vi "Buffered Log String Indicator Example.vi"() -> ()   [LabVIEW 2019, in "Logger Examples.lvlib"]
uses:
  Logger Examples.lvlib
  Source/Composed Log/Types/Log Level.ctl
  Source/String Formats/String Expression Format/String Expression Format.lvclass/String Expression Format.ctl
  Source/Composed Log/LoggerReference/LoggerReference.lvclass/LoggerReference.ctl
  601d143e-8928-4a3b-9174-3083e729aaa9.vi
  Source/String Formats/String Expression Format/Run Formatter.vi
  Source/Composed Log/LoggerReference/Return Aggregate Queues.vi
  Source/Composed Log/LoggerReference/Add Aggregate Log.vi
  601d143e-8928-4a3b-9174-3083e729aaa9.vi/16370e4d-f3cd-41c1-a9a1-4fb3403731d5.vi
  Source/Composed Log/LoggerReference/Log.vi
  Source/Composed Log/LoggerReference/Get Valid Event Time.vi
  <vilib>/dlg_ctls.llb/Space Constant.vi
  Source/Composed Log/LoggerReference/Send Add Sink.vi
  Source/Composed Log/LoggerReference/Remove Stale Logs.vi
  Source/String Formats/String Expression Format/String Expression Format.lvclass
  C:/CS/Log/Source/IStringFormat/IStringFormat.lvclass
  Source/String Control Sink/String Control Sink.lvclass
  C:/CS/Log/Source/String Log Sink/String Log Sink.lvclass
  C:/CS/Log/Source/Composed Log/Log Sink/Log Sink.lvclass
  Source/Buffered String Log Sink/Buffered String Log Sink.lvclass
  Source/Composed Log/Application Logger/Launch Worker Loop.vi
  Source/Composed Log/LoggerReference/Initialize Logger Instance.vi
  Source/Composed Log/LoggerReference/LoggerReference.lvclass
  Source/Composed Log/IErrorFormat/IErrorFormat.lvclass
  Source/Composed Log/Log Sink/Log Sink.lvclass
  Source/Composed Log/Composed Log.lvlib
panel:
  in  "Log Error":bool
  in  "Error Information":string
  in  "Error Code":i32
  in  "Event Level":T1(ring)
  out "250ms Timeout, 128 Element Buffer":string
  out "No Timeout - 50 Element Buffer":string
  out "No Timeout, Unlimited Buffer":string
  in  "Data To Log":string
  in  "Source":string="User"
  in  "Log":bool
  # "This Sink will log events as they arrive, up until the buffer is full. After that, each new event will push out the oldest."
  # "This Sink will log every event as it arrives, and grow endlessly as the application is run."
  # "This Sink will only log events on a 250ms interval. Every 250ms, if new events are available, they will be pushed to the string. A fixed length buffer is also used - only the latest 128 events will be shown."
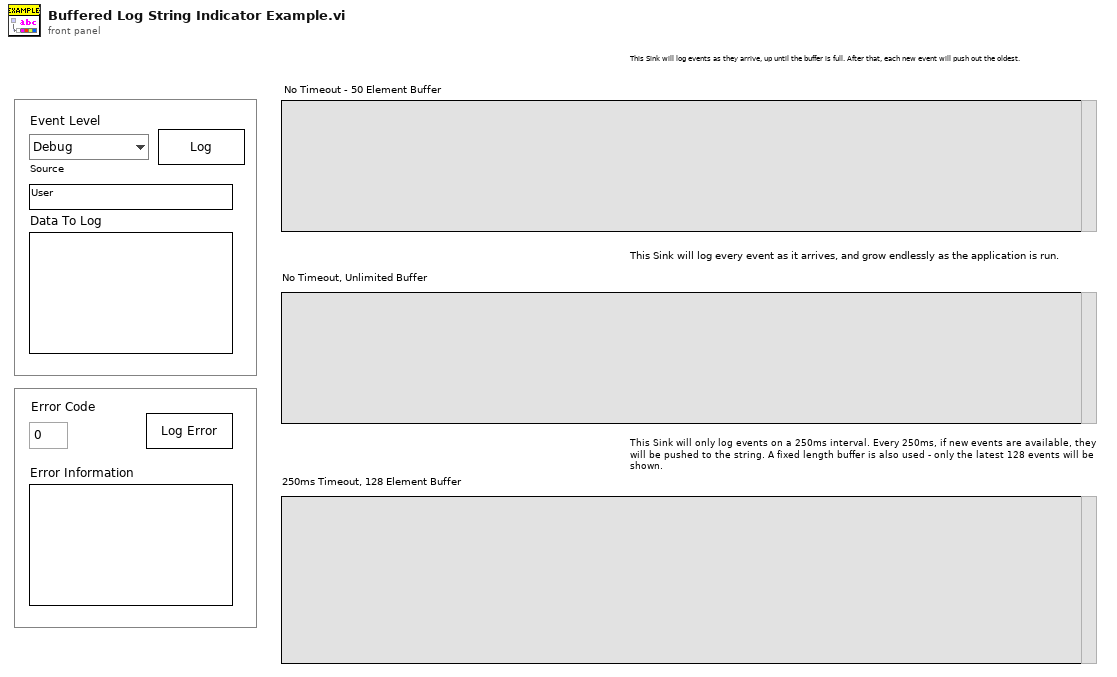
[diagram p1: front panel]
types:
  T1 = enum16{"Debug", "Info", "Warning", "Error", "Critical"}
  T2 = typedef "Composed Log.lvlib/Log Level.ctl" = enum16{"Debug", "Info", "Warning", "Error", "Critical"}
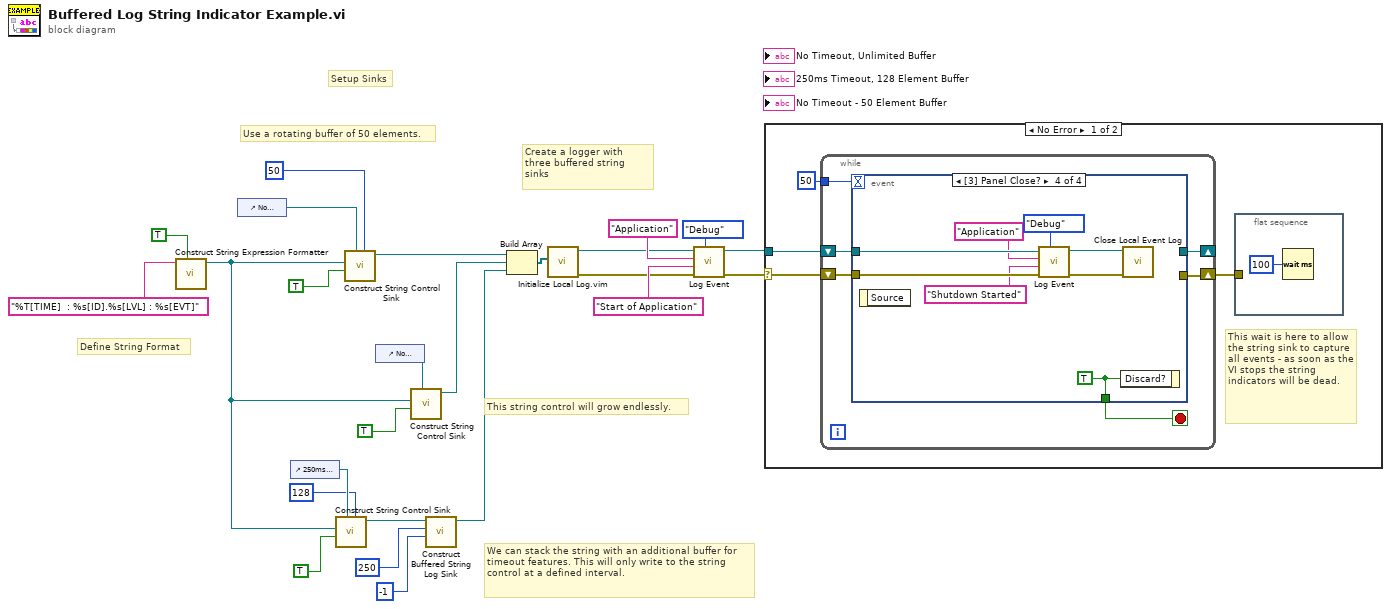
[diagram p0: block diagram]
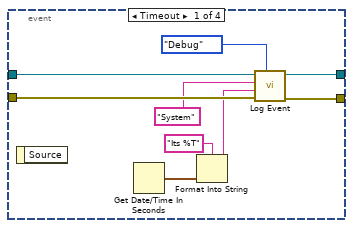
[diagram p2: hidden frame]
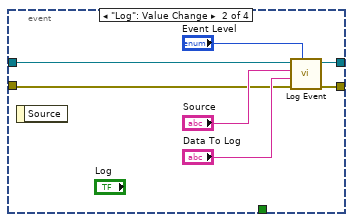
[diagram p3: hidden frame]
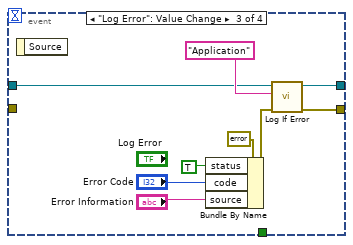
[diagram p4: hidden frame]
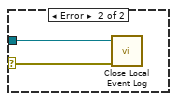
[diagram p5: hidden frame]
diagram:
  # "Use a rotating buffer of 50 elements."
  # "This string control will grow endlessly."
  # "We can stack the string with an additional buffer for timeout features. This will only write to the string control at a defined interval."
  # "Setup Sinks"
  # "Define String Format"
  # "Create a logger with three buffered string sinks"
  n1 = call "Construct String Expression Formatter.vi"("Append EOL?"=TRUE, "Format Specifier"="%T[TIME]  : %s[ID].%s[LVL] : %s[EVT]") -> ("String Expression Format out"=w1:refnum<class "String Expression Format.lvclass">)  [unwired: 8 in, 1 out]
  n2 = control-ref of="No Timeout - 50 Element Buffer"() -> (w23:refnum<vi>)
  n3 = control-ref of="250ms Timeout, 128 Element Buffer"() -> (w6:refnum<vi>)
  n4 = call "Construct String Control Sink.vi"("Buffer Length(0)"=u32 128, "Str Refnum"=w6, "AutoScroll?(F)"=TRUE, "LogFormat"=w1) -> ("String Control Sink out"=w8:refnum<class "String Control Sink.lvclass">)  [unwired: 7 in]
  n5 = call "Construct String Control Sink.vi"("Buffer Length(0)"=50, "Str Refnum"=w23, "AutoScroll?(F)"=TRUE, "LogFormat"=w1) -> ("String Control Sink out"=w11:refnum<class "String Control Sink.lvclass">)  [unwired: 7 in]
  n6 = control-ref of="No Timeout, Unlimited Buffer"() -> (w24:refnum<vi>)
  n7 = call "Construct String Control Sink.vi"("Str Refnum"=w24, "AutoScroll?(F)"=TRUE, "LogFormat"=w1) -> ("String Control Sink out"=w10:refnum<class "String Control Sink.lvclass">)  [unwired: 8 in]
  n8 = call "Construct Buffered String Log Sink.vi"("Buffer Size (128)"=-1, "Buffer Timeout ms (-1)"=250, "Sink Type"=w8) -> ("Buffered String Log Sink out"=w7:refnum<class "Buffered String Log Sink.lvclass">)  [unwired: 8 in]
  n9 = Build Array(w11, w10, w7) -> (w12:refnum<class "Log Sink.lvclass">[])
  n10 = call "Initialize Local Log.vim"("Startup Sink(s)"=w12) -> ("error out"=w18:errorcluster, "Log Instance Reference"=w17:refnum<class "LoggerReference.lvclass">)  [unwired: 8 in, 1 out]
  n11 = call "Log Event.vi"("Event Level"=Log_Level."Debug", "error in (no error)"=w18, "Data To Log"="Start of Application", "SourceID"="Application", "Log Instance"=w17) -> ("error out"=w16:errorcluster, "Log Instance Out"=w15:refnum<class "LoggerReference.lvclass">)  [unwired: 5 in]
  n12 = case shown="No Error" w16 {
    selector: w16 -> [w28 w70]
    tunnel: w15 -> [w29 w71]
    frame No Error {
      # "This wait is here to allow the string sink to capture all events - as soon as the VI stops the string indicators will be dead."
      n13 = while {
        shift-right: [w34] -> _
        shift-left: w29 -> [w35]
        shift-right: [w32] -> w26
        shift-left: w28 -> [w33]
        tunnel: 50 -> [w31]
        stop <- w36 stop-if-true
        n14 = event shown="[3] Panel Close?" {
          selector: _ -> [_ _ _ _]
          dyn-events: _ -> [_ _ _ _]
          timeout: w31 -> [_ _ _ _]
          tunnel: [_ _ _ w69] -> w36
          tunnel: w35 -> [w45 w49 w55 w67]
          tunnel: [w44 w47 w53 _] -> w34
          tunnel: w33 -> [w42 w46 _ w68]
          tunnel: [w41 w48 w54 _] -> w32
          event Timeout {
            n15 = event-data() -> ()  [unwired: 1 in, 1 out]
            n16 = Get Date/Time In Seconds() -> (seconds since 1Jan1904=w39:timestamp)
            n17 = Format Into String(format string="Its %T" ("Log Message"), w39) -> (resulting string=w37:string)  [unwired: 2 in, 1 out]
            n18 = call "Log Event.vi"("Event Level"=Log_Level."Debug", "error in (no error)"=w42, "Data To Log"=w37, "SourceID"="System" ("Event Source"), "Log Instance"=w45) -> ("error out"=w41:errorcluster, "Log Instance Out"=w44:refnum<class "LoggerReference.lvclass">)  [unwired: 5 in]
          }
          event "Log": Value Change {
            n19 = event-data() -> ()  [unwired: 1 in, 1 out]
            n20 = call "Log Event.vi"("Event Level"="Event Level", "error in (no error)"=w46, "Data To Log"="Data To Log", "SourceID"="Source", "Log Instance"=w49) -> ("error out"=w48:errorcluster, "Log Instance Out"=w47:refnum<class "LoggerReference.lvclass">)  [unwired: 5 in]
          }
          event "Log Error": Value Change {
            n21 = event-data() -> ()  [unwired: 1 in, 1 out]
            n22 = Bundle By Name(cluster=errorcluster {"status"=FALSE, "code"=0, "source"=""} ("Error In"), "status"=TRUE, "code"="Error Code", "source"="Error Information") -> (w59:errorcluster)
            n23 = call "Log If Error.vi"("Error In"=w59, "SourceID"="Application" ("Source"), "Log Instance"=w55) -> ("error out"=w54:errorcluster, "Log Instance Out"=w53:refnum<class "LoggerReference.lvclass">)  [unwired: 7 in]
          }
          event Panel Close? {
            w69 = TRUE ("Discard?")
            n24 = event-data() -> ()  [unwired: 1 in, 1 out]
            n25 = call "Log Event.vi"("Event Level"=Log_Level."Debug", "error in (no error)"=w68, "Data To Log"="Shutdown Started", "SourceID"="Application", "Log Instance"=w67) -> ("error out"=w66:errorcluster, "Log Instance Out"=w65:refnum<class "LoggerReference.lvclass">)  [unwired: 5 in]
            n26 = event-data("Discard?"=w69) -> ()  [unwired: 1 in, 1 out]
            n27 = call "Close Local Event Log.vi"("error in (no error)"=w66, "Log Instance"=w65) -> ()  [unwired: 9 in, 1 out]
          }
        }
      }
      n28 = flat-sequence {
        tunnel: w26 -> [_]
        frame #0 {
          n29 = Wait (ms)(milliseconds to wait=u32 100) -> ()  [unwired: 1 out]
        }
      }
    }
    frame Error {
      n30 = call "Close Local Event Log.vi"("error in (no error)"=w70, "Log Instance"=w71) -> ()  [unwired: 9 in, 1 out]
    }
  }
